vi "Low-Level Grab.vi"(8 "error in (no error)":errorcluster, 9 "States":T3, 11 "Session In":T1) -> (0 "error out":errorcluster, 2 "Image Out":T2, 3 "Session Out":T1)   [LabVIEW 2018]
doc: "The Grab VI acquires images continuously and displays the images in an image control using low-level acquisition VIs. A grab is appropriate for high-speed applications in which you need to process only one image at a time."
uses:
  State control.ctl
  <vilib>/userdefined/High Color/IMAQdx.ctl
  <vilib>/vision/Image Controls.llb/IMAQ Image.ctl
  <vilib>/vision/driver/IMAQdx.llb/IMAQdx Acquisition Mode.ctl
  <vilib>/vision/driver/IMAQdx.llb/IMAQdx Buffer Number Mode.ctl
  <vilib>/vision/driver/NI_Vision_Acquisition_Software.lvlib
panel:
  out "Buffer Number":u32=479
  out "Image":T2(plugin-control)
  out "Frame Rate":dbl(knob)=9.0 scale=0.0..100.0
  # "Overview: Demonstrates how to acquire continuous images from a camera using low level acquisition functions.\nRequirements: Vision Acquisition Software\nInstructions:\n1. Select the Camera Name\n2. Run the VI"
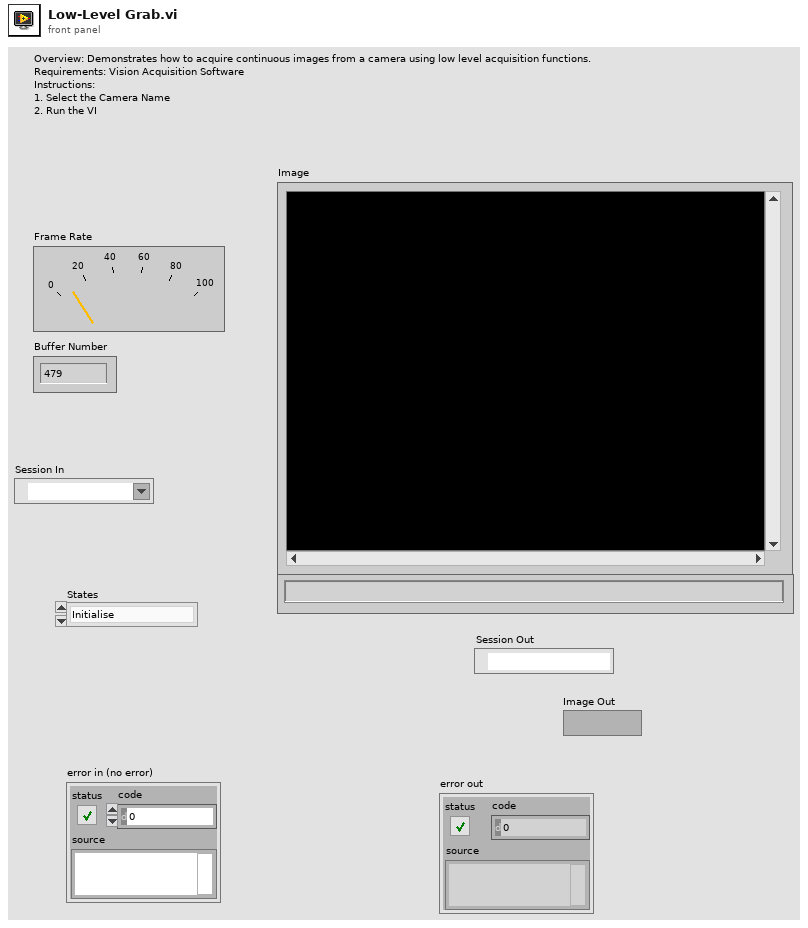
[diagram p1: front panel]
types:
  T1 = typedef "IMAQdx.ctl" = refnum<k21>
  T2 = typedef "IMAQ Image.ctl" = refnum<image>
  T3 = typedef "State control.ctl" = enum16{"Initialise", "Start camera", "Continuous Acquisition ", "Stop camera", "Dispose all"}
  T4 = typedef "NI_Vision_Acquisition_Software.lvlib/IMAQdx Acquisition Mode.ctl" = enum32{"One Shot", "Continuous"}
  T5 = typedef "NI_Vision_Acquisition_Software.lvlib/IMAQdx Buffer Number Mode.ctl" = enum32{"Next", "Last", "Buffer Number", "Every", "Last New"}
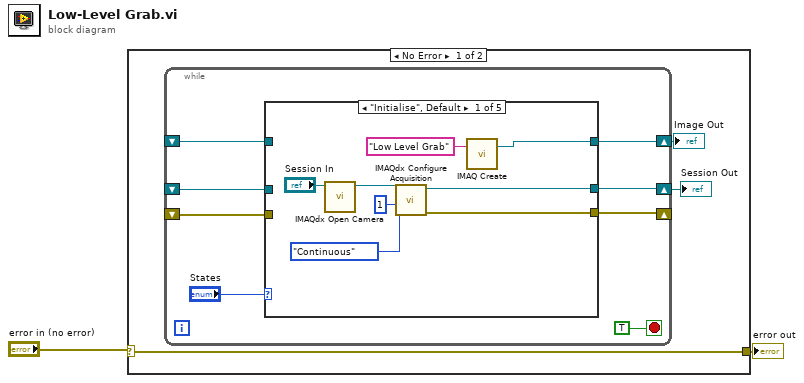
[diagram p0: block diagram]
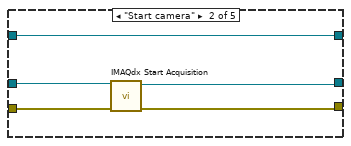
[diagram p2: hidden frame]
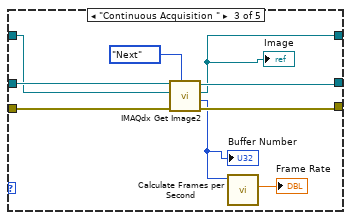
[diagram p3: hidden frame]
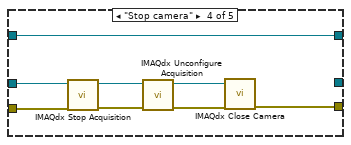
[diagram p4: hidden frame]
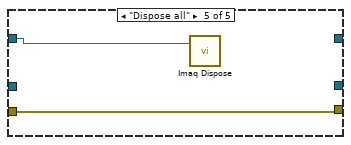
[diagram p5: hidden frame]
diagram:
  n1 = case shown="No Error" "error in (no error)" {
    selector: "error in (no error)" -> [w5 w46]
    tunnel: [w5 w46] -> w1
    frame No Error {
      n2 = while {
        shift-right: [w9] -> w4
        shift-left: _ -> [w6]
        shift-right: [w11] -> w3
        shift-left: _ -> [w8]
        shift-right: [w10] -> _
        shift-left: _ -> [w7]
        stop <- TRUE stop-if-true
        n3 = case shown="\"Initialise\", Default" "States" {
          tunnel: [w17 w23 w31 _ _] -> w11
          tunnel: [w16 w22 w30 w36 w44] -> w10
          tunnel: [w14 w24 w29 w41 _] -> w9
          tunnel: w8 -> [_ w26 w35 w43 _]
          tunnel: w7 -> [_ w25 w34 w42 w44]
          tunnel: w6 -> [_ w24 w33 w41 w45]
          frame "Initialise", Default {
            n4 = call <vilib>:"IMAQdx Open Camera.vi"("Session In"="Session In") -> ("Session Out"=w18:T1)  [unwired: 9 in, 1 out]
            n5 = call <vilib>:"IMAQdx Configure Acquisition.vi"("Number of Buffers"=u32 1, "Continuous?"=IMAQdx_Acquisition_Mode."Continuous", "Session In"=w18) -> ("error out"=w16:errorcluster, "Session Out"=w17:T1)  [unwired: 7 in]
            n6 = call "IMAQ Create"("Image Name"="Low Level Grab") -> ("New Image"=w14:T2)  [unwired: 3 in, 2 out]
          }
          frame "Start camera" {
            n7 = call <vilib>:"IMAQdx Start Acquisition.vi"("error in"=w25, "Session In"=w26) -> ("error out"=w22:errorcluster, "Session Out"=w23:T1)  [unwired: 8 in]
          }
          frame "Continuous Acquisition " {
            n8 = call <vilib>:"IMAQdx Get Image2.vi"("Buffer Number Mode (Next)"=IMAQdx_Buffer_Number_Mode."Next", "error in"=w34, "Image In"=w33, "Session In"=w35) -> ("error out"=w30:errorcluster, "Buffer Number Out"=w27:u32, "Image Out"=w29:T2, "Session Out"=w31:T1)  [unwired: 4 in]
            "Image" <- w29
            "Buffer Number" <- w27
            n9 = call <vilib>:"Calculate Frames per Second.vi"("Buffer Number"=w27) -> ("Processed Frames/s"=→"Frame Rate":dbl)  [unwired: 8 in, 2 out]
          }
          frame "Stop camera" {
            n10 = call <vilib>:"IMAQdx Stop Acquisition.vi"("error in"=w42, "Session In"=w43) -> ("error out"=w39:errorcluster, "Session Out"=w40:T1)  [unwired: 8 in]
            n11 = call <vilib>:"IMAQdx Unconfigure Acquisition.vi"("error in"=w39, "Session In"=w40) -> ("error out"=w37:errorcluster, "Session Out"=w38:T1)  [unwired: 8 in]
            n12 = call <vilib>:"IMAQdx Close Camera.vi"("error in"=w37, "Session In"=w38) -> ("error out"=w36:errorcluster)  [unwired: 9 in]
          }
          frame "Dispose all" {
            n13 = call "Imaq Dispose"("Image"=w45) -> ()  [unwired: 5 in, 1 out]
          }
        }
      }
      "Image Out" <- w4
      "Session Out" <- w3
    }
    frame Error {
    }
  }
  "error out" <- w1
